vi "Write Scalar Data.vi"(8 "error in (no error)":errorcluster, 9 "Changed?":bool[](array[boolean]), 10 "Values":dbl[](array[numeric]), 11 "Cluster":T1 {"Data Type" format="%.0x"}) -> (0 "error out":errorcluster, 2 "Values":dbl[](array[numeric]), 3 "Cluster":T1 {"Data Type" format="%.0x"})   [LabVIEW 2016, in "FPGA Addon Engine.lvlib"]
uses:
  FPGA Addon Engine.lvlib
  Types/Register Settings.ctl
  Shared/Data Type.ctl
  Shared/Scalar Type.ctl
  <vilib>/rvi/errors/niLvFpgaAdjustHostInterfaceError.vi
  <vilib>/Utility/error.llb/Error Cluster From Error Code.vi
  <vilib>/rvi/interface/nirviReadWriteControl/nirviReadWriteControl.xnode
  <vilib>/rvi/interface/Simulation/niFpgaSimulationCallBeginRW.vi
  NiFpgaLv.dll
  Shared/FPGA Addon Shared.lvlib
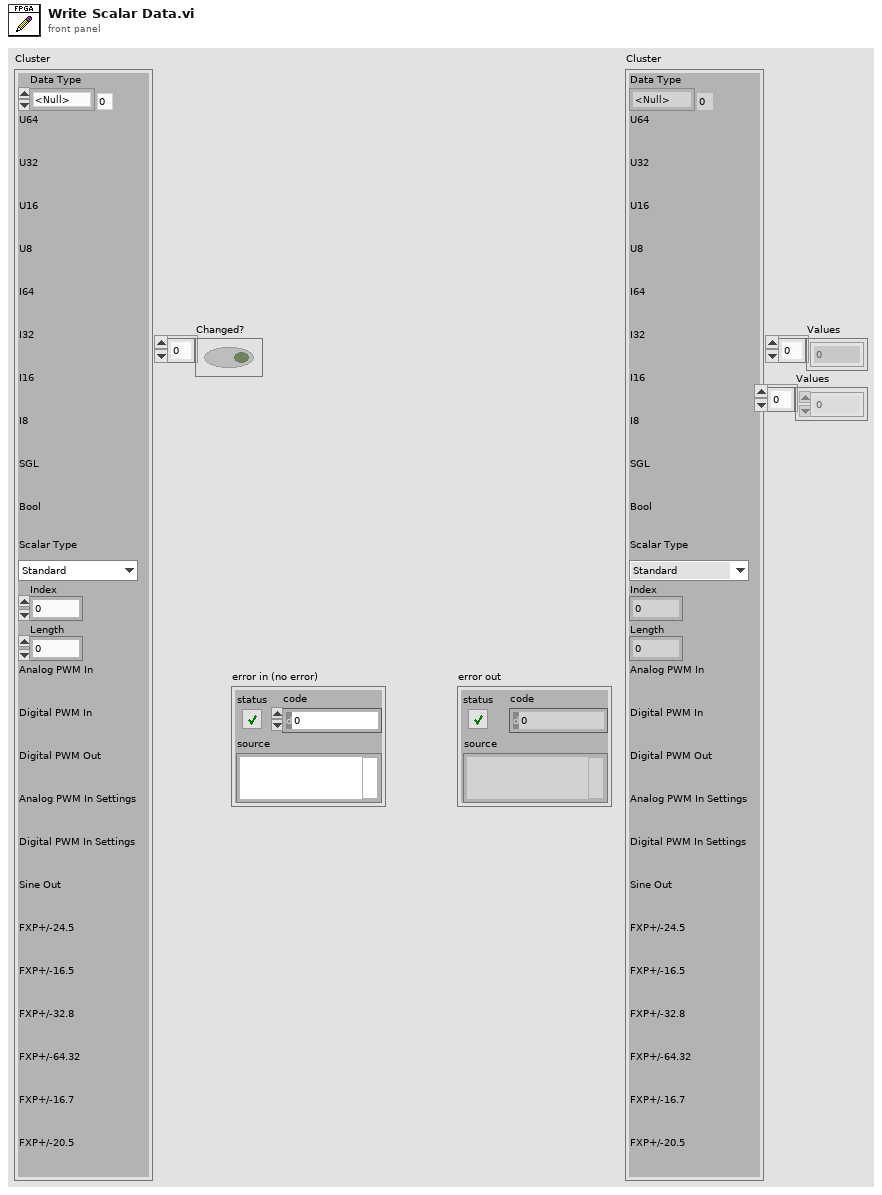
[diagram p1: front panel]
types:
  T1 = typedef "FPGA Addon Engine.lvlib/Register Settings.ctl" = cluster{"Data Type":T2, "U64":refnum<k20>, "U32":refnum<k20>, "U16":refnum<k20>, "U8":refnum<k20>, "I64":refnum<k20>, "I32":refnum<k20>, "I16":refnum<k20>, "I8":refnum<k20>, "SGL":refnum<k20>, "Bool":refnum<k20>, "Scalar Type":T3, "Index":i32, "Length":i32, "Analog PWM In":refnum<k20>, "Digital PWM In":refnum<k20>, "Digital PWM Out":refnum<k20>, "Analog PWM In Settings":refnum<k20>, "Digital PWM In Settings":refnum<k20>, "Sine Out":refnum<k20>, "FXP+/-24.5":refnum<k20>, "FXP+/-16.5":refnum<k20>, "FXP+/-32.8":refnum<k20>, "FXP+/-64.32":refnum<k20>, "FXP+/-16.7":refnum<k20>, "FXP+/-20.5":refnum<k20>}
  T2 = typedef "FPGA Addon Shared.lvlib/Data Type.ctl" = enum8{"<Null>", "I8", "I16", "I32", "I64", "U8", "U16", "U32", "U64", "SGL", "Boolean", "Analog PWM In Settings", "Analog PWM In", "Digital PWM In Settings", "Digital PWM In", "Digital PWM Out", "Sine Out", "FXP+/-24.5", "FXP+/-16.5", "FXP+/-32.8", "FXP+/-64.32", "FXP+/-16.7", "FXP+/-20.5"}
  T3 = typedef "FPGA Addon Shared.lvlib/Scalar Type.ctl" = enum16{"Standard", "Bitpacked"}
  T4 = cluster{"ACTIVE EDGE":bool, "TIMEOUT":u32, "THRESHOLD":fxp<+/-,32,8>}
  T5 = cluster{"ACTIVE EDGE":bool, "ACTIVE TICKS":u32, "INACTIVE TICKS":u32}
  T6 = cluster{"AMP":fxp<+/-,32,8>, "OFFSET":fxp<+/-,32,8>, "PERIODS/TICKS":fxp<+,32,0>}
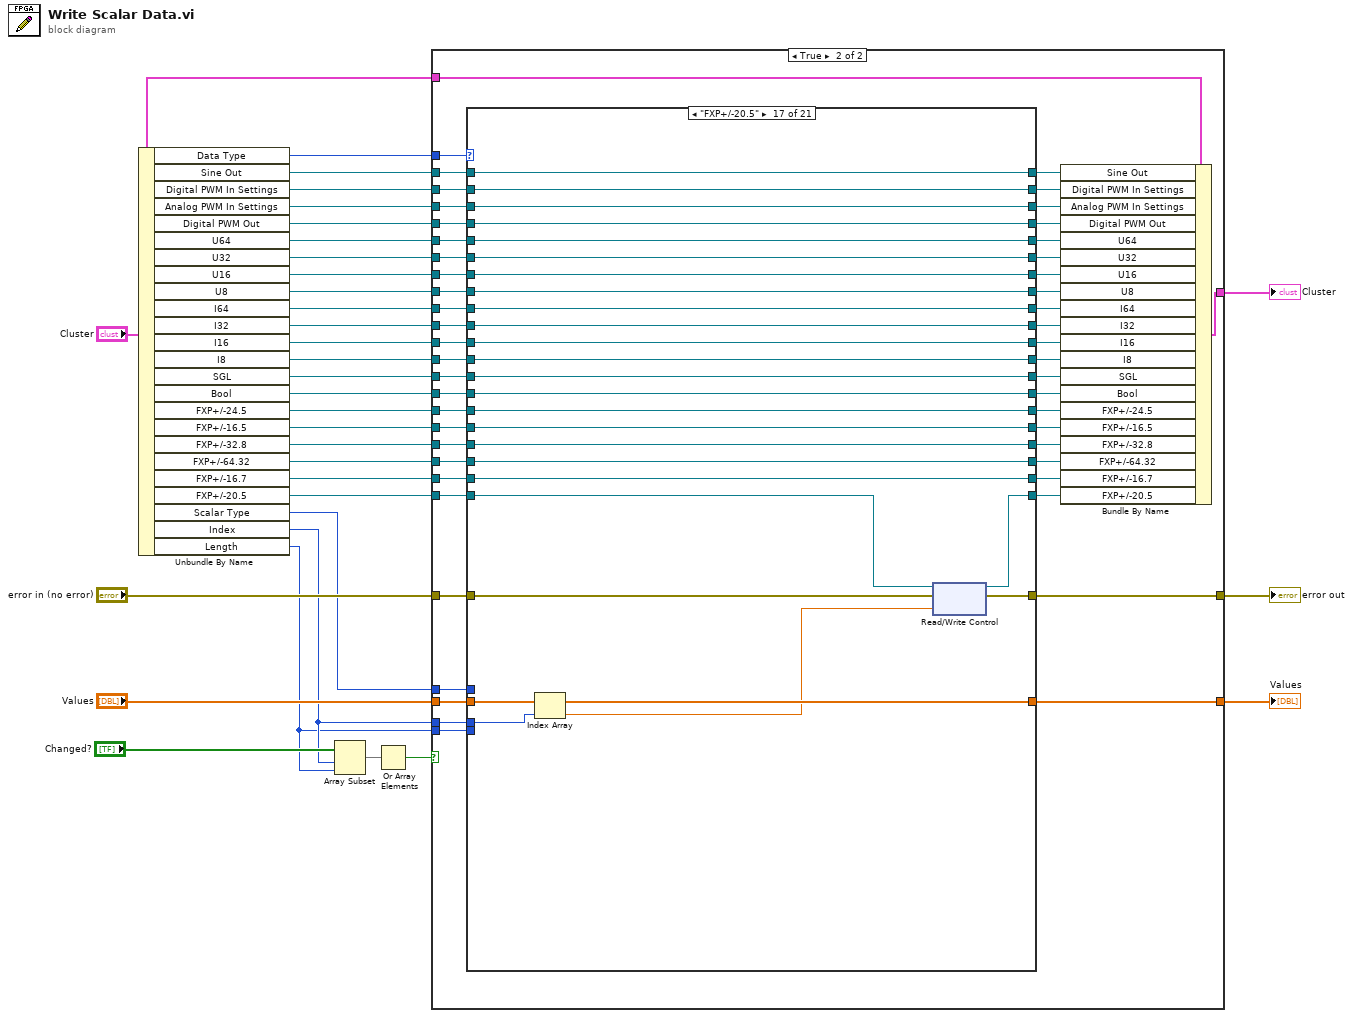
[diagram p0: block diagram]
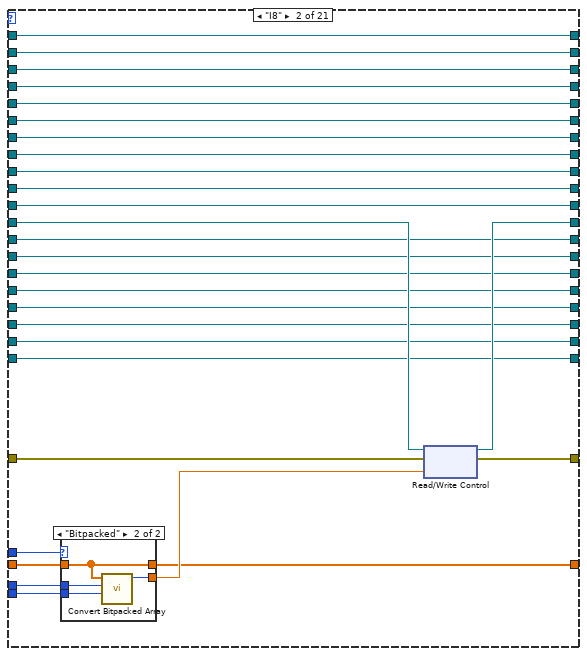
[diagram p4: hidden frame]
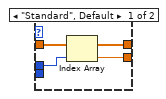
[diagram p5: hidden frame]
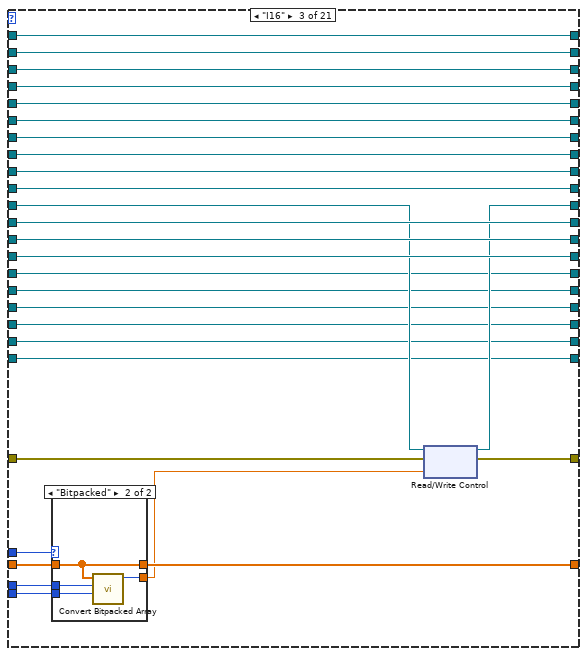
[diagram p6: hidden frame]
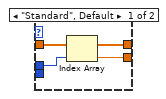
[diagram p7: hidden frame]
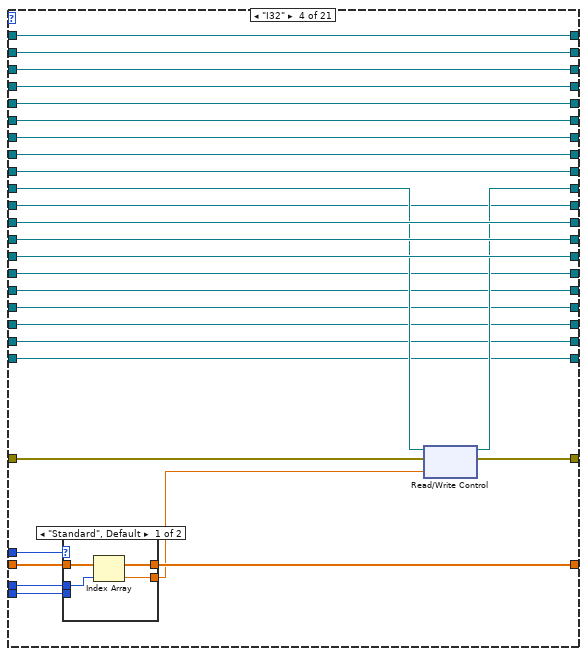
[diagram p8: hidden frame]
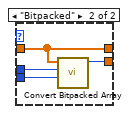
[diagram p9: hidden frame]
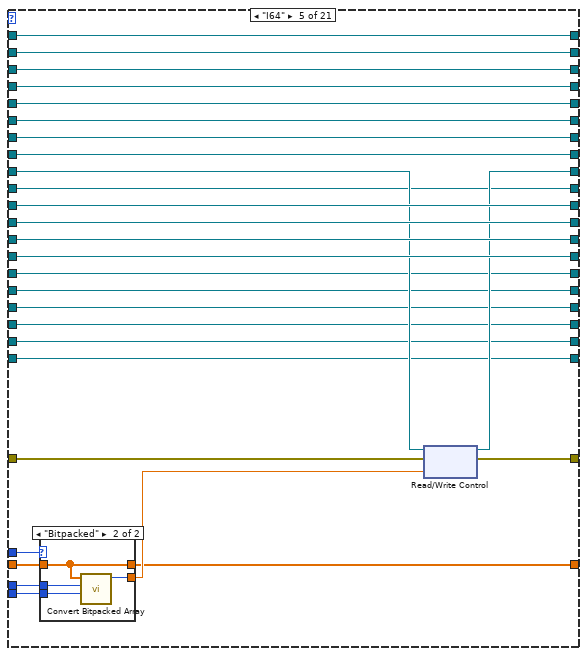
[diagram p10: hidden frame]
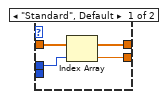
[diagram p11: hidden frame]
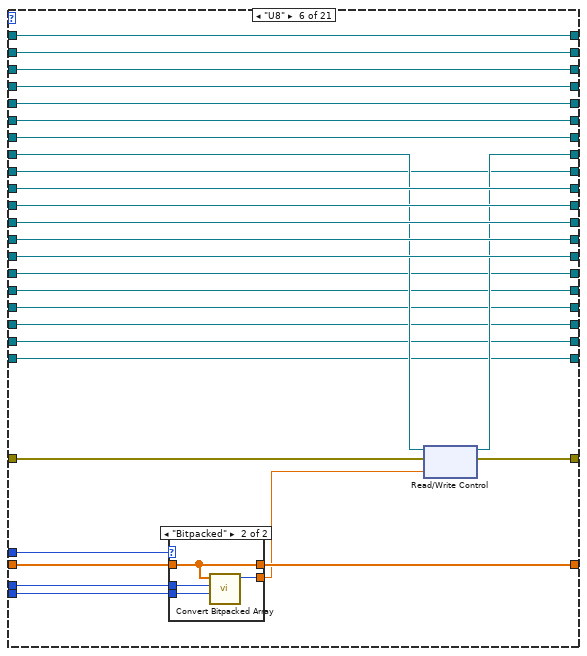
[diagram p12: hidden frame]
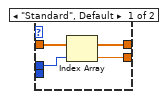
[diagram p13: hidden frame]
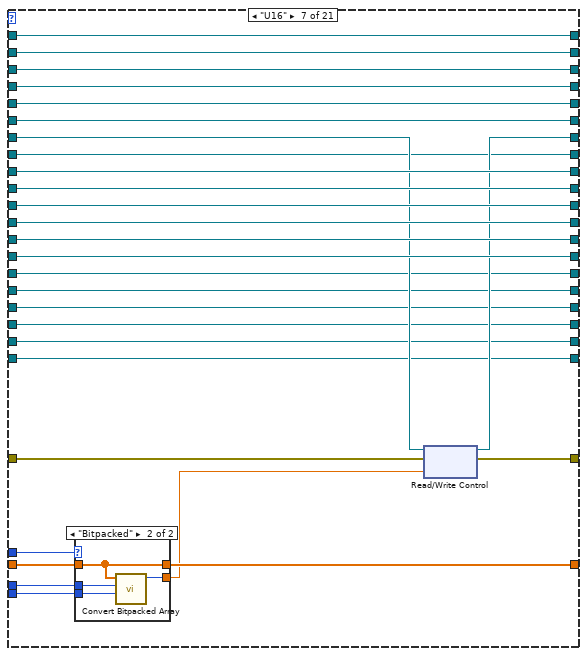
[diagram p14: hidden frame]
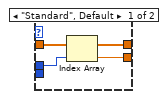
[diagram p15: hidden frame]
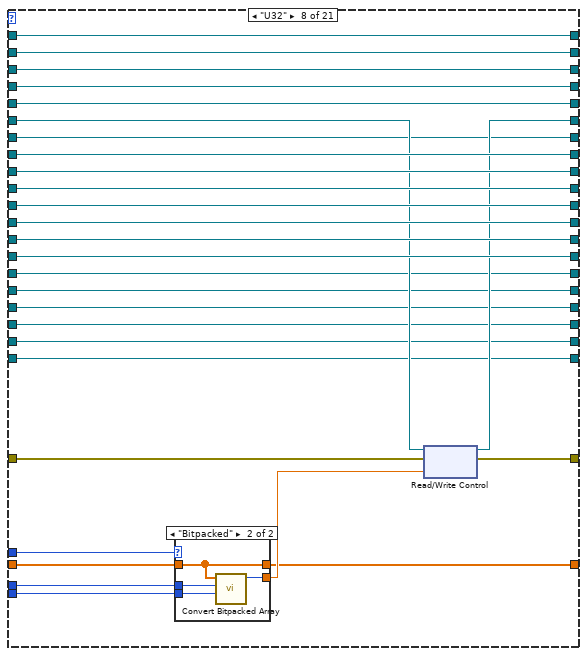
[diagram p16: hidden frame]
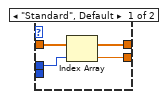
[diagram p17: hidden frame]
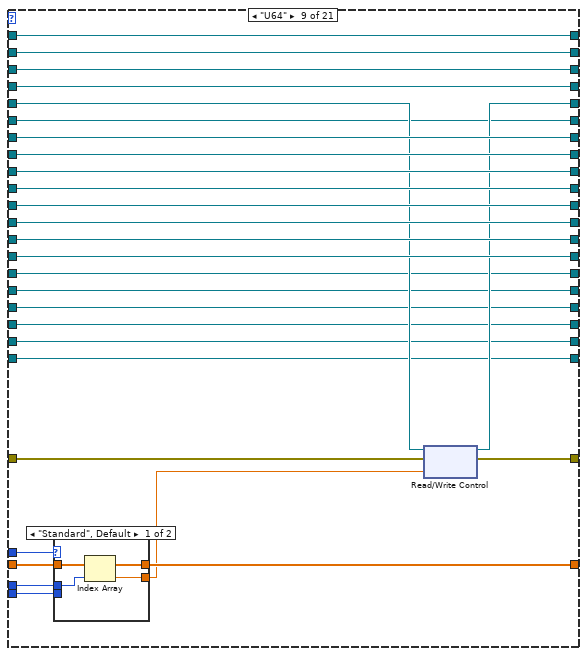
[diagram p18: hidden frame]
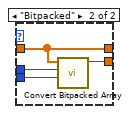
[diagram p19: hidden frame]
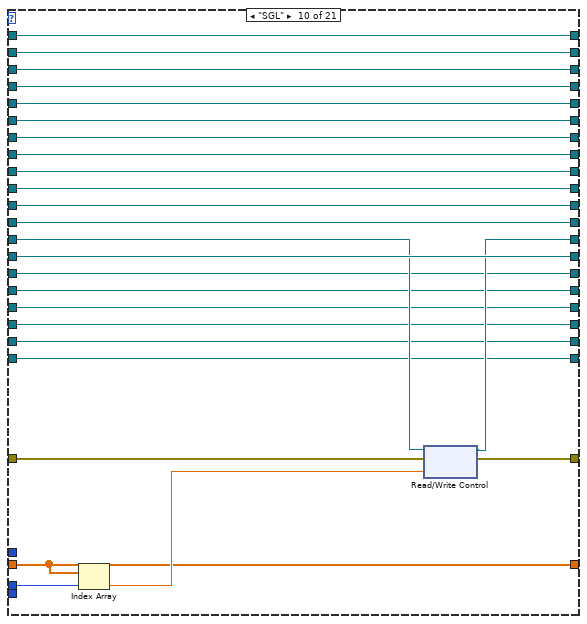
[diagram p20: hidden frame]
diagram:
  n1 = Unbundle By Name("Cluster") -> ("Data Type"=w33:T2, "Sine Out"=w7:refnum<k20>, "Digital PWM In Settings"=w13:refnum<k20>, "Analog PWM In Settings"=w14:refnum<k20>, "Digital PWM Out"=w15:refnum<k20>, "U64"=w20:refnum<k20>, "U32"=w21:refnum<k20>, "U16"=w22:refnum<k20>, "U8"=w23:refnum<k20>, "I64"=w24:refnum<k20>, "I32"=w25:refnum<k20>, "I16"=w26:refnum<k20>, "I8"=w32:refnum<k20>, "SGL"=w28:refnum<k20>, "Bool"=w27:refnum<k20>, "FXP+/-24.5"=w3:refnum<k20>, "FXP+/-16.5"=w4:refnum<k20>, "FXP+/-32.8"=w5:refnum<k20>, "FXP+/-64.32"=w6:refnum<k20>, "FXP+/-16.7"=w2:refnum<k20>, "FXP+/-20.5"=w1:refnum<k20>, "Scalar Type"=w16:T3, "Index"=w11:i32, "Length"=w10:i32)
  n2 = Array Subset(array="Changed?", index=w11, length=w10) -> (w9:bool[])
  n3 = Or Array Elements(Boolean array=w9) -> (logical OR=w8:bool)
  n4 = case shown="True" w8 {
    tunnel: w33 -> [_ w86]
    tunnel: w32 -> [_ w85]
    tunnel: "error in (no error)" -> [w35 w84]
    tunnel: [w35 w83] -> w30
    tunnel: "Cluster" -> [w36 w82]
    tunnel: w28 -> [_ w79]
    tunnel: w27 -> [_ w78]
    tunnel: w26 -> [_ w75]
    tunnel: w25 -> [_ w73]
    tunnel: w24 -> [_ w71]
    tunnel: w23 -> [_ w69]
    tunnel: w22 -> [_ w67]
    tunnel: w21 -> [_ w65]
    tunnel: w20 -> [_ w63]
    tunnel: [w36 w62] -> w19
    tunnel: [w34 w61] -> w18
    tunnel: "Values" -> [w34 w60]
    tunnel: w16 -> [_ w59]
    tunnel: w15 -> [_ w57]
    tunnel: w14 -> [_ w56]
    tunnel: w13 -> [_ w53]
    tunnel: w11 -> [_ w52]
    tunnel: w10 -> [_ w51]
    tunnel: w7 -> [_ w50]
    tunnel: w6 -> [_ w47]
    tunnel: w5 -> [_ w46]
    tunnel: w4 -> [_ w43]
    tunnel: w3 -> [_ w42]
    tunnel: w2 -> [_ w40]
    tunnel: w1 -> [_ w38]
    frame False {
    }
    frame True {
      n5 = case shown="\"FXP+/-20.5\"" w86 {
        tunnel: w85 -> [w106 w137 w163 w200 w237 w274 w311 w348 w385 w419 w448 w474 w500 w526 w552 w578 w604 w631 w665 w722 w759]
        tunnel: w84 -> [w98 w136 w173 w209 w245 w281 w317 w353 w389 w422 w450 w476 w502 w528 w554 w580 w606 w628 w662 w710 w747]
        tunnel: [w98 w135 w172 w208 w244 w280 w316 w352 w388 w421 w449 w475 w501 w527 w553 w579 w605 w627 w661 w709 w746] -> w83
        tunnel: [w106 w134 w163 w200 w237 w274 w311 w348 w385 w419 w448 w474 w500 w526 w552 w578 w604 w631 w665 w722 w759] -> w81
        tunnel: [w107 w133 w171 w207 w243 w279 w315 w351 w387 w410 w438 w466 w492 w518 w544 w570 w596 w630 w664 w721 w758] -> w80
        tunnel: w79 -> [w107 w133 w171 w207 w243 w279 w315 w351 w387 w412 w438 w466 w492 w518 w544 w570 w596 w630 w664 w721 w758]
        tunnel: w78 -> [w108 w132 w170 w206 w242 w278 w314 w350 w386 w420 w440 w455 w482 w509 w536 w562 w589 w629 w663 w720 w757]
        tunnel: [w108 w132 w170 w206 w242 w278 w314 w350 w386 w420 w439 w455 w482 w509 w536 w562 w589 w629 w663 w720 w757] -> w77
        tunnel: [w105 w131 w161 w197 w236 w273 w310 w347 w384 w418 w447 w473 w499 w525 w551 w577 w603 w632 w666 w719 w756] -> w76
        tunnel: w75 -> [w105 w131 w162 w197 w236 w273 w310 w347 w384 w418 w447 w473 w499 w525 w551 w577 w603 w632 w666 w719 w756]
        tunnel: [w104 w130 w169 w198 w233 w272 w309 w346 w383 w417 w446 w472 w498 w524 w550 w576 w602 w633 w667 w718 w755] -> w74
        tunnel: w73 -> [w104 w130 w169 w199 w233 w272 w309 w346 w383 w417 w446 w472 w498 w524 w550 w576 w602 w633 w667 w718 w755]
        tunnel: [w103 w129 w168 w205 w234 w269 w308 w345 w382 w416 w445 w471 w497 w523 w549 w575 w601 w634 w668 w717 w754] -> w72
        tunnel: w71 -> [w103 w129 w168 w205 w235 w269 w308 w345 w382 w416 w445 w471 w497 w523 w549 w575 w601 w634 w668 w717 w754]
        tunnel: [w102 w128 w167 w204 w241 w270 w305 w344 w381 w415 w444 w470 w496 w522 w548 w574 w600 w635 w669 w716 w753] -> w70
        tunnel: w69 -> [w102 w128 w167 w204 w241 w271 w305 w344 w381 w415 w444 w470 w496 w522 w548 w574 w600 w635 w669 w716 w753]
        tunnel: [w101 w127 w166 w203 w240 w277 w306 w341 w380 w414 w443 w469 w495 w521 w547 w573 w599 w636 w670 w715 w752] -> w68
        tunnel: w67 -> [w101 w127 w166 w203 w240 w277 w307 w341 w380 w414 w443 w469 w495 w521 w547 w573 w599 w636 w670 w715 w752]
        tunnel: [w100 w126 w165 w202 w239 w276 w313 w342 w377 w413 w442 w468 w494 w520 w546 w572 w598 w637 w671 w714 w751] -> w66
        tunnel: w65 -> [w100 w126 w165 w202 w239 w276 w313 w343 w377 w413 w442 w468 w494 w520 w546 w572 w598 w637 w671 w714 w751]
        tunnel: [w99 w125 w164 w201 w238 w275 w312 w349 w378 w411 w441 w467 w493 w519 w545 w571 w597 w638 w672 w713 w750] -> w64
        tunnel: w63 -> [w99 w125 w164 w201 w238 w275 w312 w349 w379 w411 w441 w467 w493 w519 w545 w571 w597 w638 w672 w713 w750]
        tunnel: [w97 w119 w156 w192 w227 w264 w300 w335 w372 w407 w435 w465 w491 w517 w543 w569 w595 w622 w658 w703 w745] -> w61
        tunnel: w60 -> [w97 w124 w160 w196 w232 w268 w304 w340 w376 w407 w435 w465 w491 w517 w543 w569 w595 w622 w658 w703 w745]
        tunnel: w51 -> [_ w122 w158 w193 w229 w267 w302 w338 w373 _ _ _ _ _ _ _ _ w623 w659 w702 w744]
        tunnel: w59 -> [_ w121 w157 w195 w231 w265 w301 w337 w375 _ _ _ _ _ _ _ _ _ _ _ _]
        tunnel: w52 -> [_ w123 w159 w194 w230 w266 w303 w339 w374 w409 w434 w464 w490 w516 w542 w568 w594 w624 w660 w701 w743]
        tunnel: [w96 w116 w152 w188 w224 w260 w296 w332 w368 w404 w430 w461 w487 w513 w539 w565 w591 w640 w673 w707 w739] -> w58
        tunnel: w57 -> [w96 w116 w152 w188 w224 w260 w296 w332 w368 w404 w430 w461 w487 w513 w539 w565 w591 w640 w673 w708 w739]
        tunnel: w56 -> [w95 w117 w153 w189 w225 w261 w297 w333 w369 w405 w431 w462 w488 w514 w540 w566 w592 w626 w652 w712 w749]
        tunnel: [w95 w117 w153 w189 w225 w261 w297 w333 w369 w405 w431 w462 w488 w514 w540 w566 w592 w625 w652 w712 w749] -> w55
        tunnel: [w94 w118 w154 w190 w226 w262 w298 w334 w370 w406 w432 w463 w489 w515 w541 w567 w593 w639 w654 w711 w748] -> w54
        tunnel: w53 -> [w94 w118 w154 w190 w226 w262 w298 w334 w370 w406 w432 w463 w489 w515 w541 w567 w593 w639 w653 w711 w748]
        tunnel: w50 -> [w93 w115 w151 w187 w223 w259 w295 w331 w367 w403 w429 w460 w486 w512 w538 w564 w590 w615 w649 w682 w741]
        tunnel: [w93 w115 w151 w187 w223 w259 w295 w331 w367 w403 w429 w460 w486 w512 w538 w564 w590 w615 w649 w682 w740] -> w49
        tunnel: [w92 w114 w150 w186 w222 w258 w294 w330 w366 w402 w428 w459 w485 w511 w531 w558 w585 w614 w646 w679 w731] -> w48
        tunnel: w47 -> [w92 w114 w150 w186 w222 w258 w294 w330 w366 w402 w428 w459 w485 w511 w533 w558 w585 w614 w646 w679 w731]
        tunnel: w46 -> [w91 w113 w149 w185 w221 w257 w293 w329 w365 w401 w427 w458 w484 w505 w532 w559 w586 w613 w645 w678 w730]
        tunnel: [w91 w113 w149 w185 w221 w257 w293 w329 w365 w401 w427 w458 w484 w506 w532 w559 w586 w613 w645 w678 w730] -> w45
        tunnel: [w90 w112 w148 w184 w220 w256 w292 w328 w364 w400 w426 w457 w479 w507 w534 w560 w587 w612 w644 w677 w729] -> w44
        tunnel: w43 -> [w90 w112 w148 w184 w220 w256 w292 w328 w364 w400 w426 w457 w480 w507 w534 w560 w587 w612 w644 w677 w729]
        tunnel: w42 -> [w89 w111 w147 w183 w219 w255 w291 w327 w363 w399 w425 w454 w481 w508 w535 w561 w588 w611 w643 w676 w728]
        tunnel: [w89 w111 w147 w183 w219 w255 w291 w327 w363 w399 w425 w453 w481 w508 w535 w561 w588 w611 w643 w676 w728] -> w41
        tunnel: w40 -> [w88 w110 w146 w182 w218 w254 w290 w326 w362 w398 w424 w452 w478 w504 w530 w557 w583 w610 w642 w675 w727]
        tunnel: [w88 w110 w146 w182 w218 w254 w290 w326 w362 w398 w424 w452 w478 w504 w530 w556 w583 w610 w642 w675 w727] -> w39
        tunnel: w38 -> [w87 w109 w145 w181 w217 w253 w289 w325 w361 w397 w423 w451 w477 w503 w529 w555 w584 w607 w641 w674 w726]
        tunnel: [w87 w109 w145 w181 w217 w253 w289 w325 w361 w397 w423 w451 w477 w503 w529 w555 w582 w607 w641 w674 w726] -> w37
        frame "<Null>", Default {
        }
        frame "I8" {
          n6 = case shown="\"Bitpacked\"" w121 {
            tunnel: w124 -> [w138 w141]
            tunnel: w123 -> [w140 w144]
            tunnel: [w139 w142] -> w120
            tunnel: w122 -> [_ w143]
            tunnel: [w138 w141] -> w119
            frame "Standard", Default {
              n7 = Index Array(array=w138, index=w140) -> (element=w139:dbl)
            }
            frame "Bitpacked" {
              n8 = call "Convert Bitpacked Array.vi"("Length"=w143, "Index"=w144, "Values"=w141) -> ("Numeric"=w142:u64)  [unwired: 8 in]
            }
          }
          n9 = xnode "Read/Write Control"("FPGA VI Reference In"=w137, "error in"=w136, "Value"=w120) -> ("FPGA VI Reference Out"=w134:refnum<k20>, "error out"=w135:errorcluster)
        }
        frame "I16" {
          n10 = case shown="\"Bitpacked\"" w157 {
            tunnel: w160 -> [w174 w177]
            tunnel: w159 -> [w176 w180]
            tunnel: [w175 w178] -> w155
            tunnel: w158 -> [_ w179]
            tunnel: [w174 w177] -> w156
            frame "Standard", Default {
              n11 = Index Array(array=w174, index=w176) -> (element=w175:dbl)
            }
            frame "Bitpacked" {
              n12 = call "Convert Bitpacked Array.vi"("Length"=w179, "Index"=w180, "Values"=w177) -> ("Numeric"=w178:u64)  [unwired: 8 in]
            }
          }
          n13 = xnode "Read/Write Control"("FPGA VI Reference In"=w162, "error in"=w173, "Value"=w155) -> ("FPGA VI Reference Out"=w161:refnum<k20>, "error out"=w172:errorcluster)
        }
        frame "I32" {
          n14 = case shown="\"Standard\", Default" w195 {
            tunnel: w196 -> [w210 w213]
            tunnel: w194 -> [w212 w216]
            tunnel: [w211 w214] -> w191
            tunnel: w193 -> [_ w215]
            tunnel: [w210 w213] -> w192
            frame "Standard", Default {
              n15 = Index Array(array=w210, index=w212) -> (element=w211:dbl)
            }
            frame "Bitpacked" {
              n16 = call "Convert Bitpacked Array.vi"("Length"=w215, "Index"=w216, "Values"=w213) -> ("Numeric"=w214:u64)  [unwired: 8 in]
            }
          }
          n17 = xnode "Read/Write Control"("FPGA VI Reference In"=w199, "error in"=w209, "Value"=w191) -> ("FPGA VI Reference Out"=w198:refnum<k20>, "error out"=w208:errorcluster)
        }
        frame "I64" {
          n18 = case shown="\"Bitpacked\"" w231 {
            tunnel: w232 -> [w246 w249]
            tunnel: w230 -> [w248 w252]
            tunnel: [w247 w250] -> w228
            tunnel: w229 -> [_ w251]
            tunnel: [w246 w249] -> w227
            frame "Standard", Default {
              n19 = Index Array(array=w246, index=w248) -> (element=w247:dbl)
            }
            frame "Bitpacked" {
              n20 = call "Convert Bitpacked Array.vi"("Length"=w251, "Index"=w252, "Values"=w249) -> ("Numeric"=w250:u64)  [unwired: 8 in]
            }
          }
          n21 = xnode "Read/Write Control"("FPGA VI Reference In"=w235, "error in"=w245, "Value"=w228) -> ("FPGA VI Reference Out"=w234:refnum<k20>, "error out"=w244:errorcluster)
        }
        frame "U8" {
          n22 = case shown="\"Bitpacked\"" w265 {
            tunnel: w268 -> [w282 w285]
            tunnel: w266 -> [w284 w288]
            tunnel: [w283 w286] -> w263
            tunnel: w267 -> [_ w287]
            tunnel: [w282 w285] -> w264
            frame "Standard", Default {
              n23 = Index Array(array=w282, index=w284) -> (element=w283:dbl)
            }
            frame "Bitpacked" {
              n24 = call "Convert Bitpacked Array.vi"("Length"=w287, "Index"=w288, "Values"=w285) -> ("Numeric"=w286:u64)  [unwired: 8 in]
            }
          }
          n25 = xnode "Read/Write Control"("FPGA VI Reference In"=w271, "error in"=w281, "Value"=w263) -> ("FPGA VI Reference Out"=w270:refnum<k20>, "error out"=w280:errorcluster)
        }
        frame "U16" {
          n26 = case shown="\"Bitpacked\"" w301 {
            tunnel: w304 -> [w318 w321]
            tunnel: w303 -> [w320 w324]
            tunnel: [w319 w322] -> w299
            tunnel: w302 -> [_ w323]
            tunnel: [w318 w321] -> w300
            frame "Standard", Default {
              n27 = Index Array(array=w318, index=w320) -> (element=w319:dbl)
            }
            frame "Bitpacked" {
              n28 = call "Convert Bitpacked Array.vi"("Length"=w323, "Index"=w324, "Values"=w321) -> ("Numeric"=w322:u64)  [unwired: 8 in]
            }
          }
          n29 = xnode "Read/Write Control"("FPGA VI Reference In"=w307, "error in"=w317, "Value"=w299) -> ("FPGA VI Reference Out"=w306:refnum<k20>, "error out"=w316:errorcluster)
        }
        frame "U32" {
          n30 = case shown="\"Bitpacked\"" w337 {
            tunnel: w340 -> [w354 w357]
            tunnel: w339 -> [w356 w360]
            tunnel: [w355 w358] -> w336
            tunnel: w338 -> [_ w359]
            tunnel: [w354 w357] -> w335
            frame "Standard", Default {
              n31 = Index Array(array=w354, index=w356) -> (element=w355:dbl)
            }
            frame "Bitpacked" {
              n32 = call "Convert Bitpacked Array.vi"("Length"=w359, "Index"=w360, "Values"=w357) -> ("Numeric"=w358:u64)  [unwired: 8 in]
            }
          }
          n33 = xnode "Read/Write Control"("FPGA VI Reference In"=w343, "error in"=w353, "Value"=w336) -> ("FPGA VI Reference Out"=w342:refnum<k20>, "error out"=w352:errorcluster)
        }
        frame "U64" {
          n34 = case shown="\"Standard\", Default" w375 {
            tunnel: w376 -> [w390 w393]
            tunnel: w374 -> [w392 w396]
            tunnel: [w391 w394] -> w371
            tunnel: w373 -> [_ w395]
            tunnel: [w390 w393] -> w372
            frame "Standard", Default {
              n35 = Index Array(array=w390, index=w392) -> (element=w391:dbl)
            }
            frame "Bitpacked" {
              n36 = call "Convert Bitpacked Array.vi"("Length"=w395, "Index"=w396, "Values"=w393) -> ("Numeric"=w394:u64)  [unwired: 8 in]
            }
          }
          n37 = xnode "Read/Write Control"("FPGA VI Reference In"=w379, "error in"=w389, "Value"=w371) -> ("FPGA VI Reference Out"=w378:refnum<k20>, "error out"=w388:errorcluster)
        }
        frame "SGL" {
          n38 = Index Array(array=w407, index=w409) -> (element=w408:dbl)
          n39 = xnode "Read/Write Control"("FPGA VI Reference In"=w412, "error in"=w422, "Value"=w408) -> ("FPGA VI Reference Out"=w410:refnum<k20>, "error out"=w421:errorcluster)
        }
        frame "Boolean" {
          n40 = Index Array(array=w435, index=w434) -> (element=w433:dbl)
          n41 = To Unsigned Byte Integer(number=w433) -> (unsigned 8bit integer=w436:u8)
          n42 = Greater Than 0?(x=w436) -> (x > 0?=w437:bool)
          n43 = xnode "Read/Write Control"("FPGA VI Reference In"=w440, "error in"=w450, "Value"=w437) -> ("FPGA VI Reference Out"=w439:refnum<k20>, "error out"=w449:errorcluster)
        }
        frame "FXP+/-24.5" {
          n44 = Index Array(array=w465, index=w464) -> (element=w456:dbl)
          n45 = xnode "Read/Write Control"("FPGA VI Reference In"=w454, "error in"=w476, "Value"=w456) -> ("FPGA VI Reference Out"=w453:refnum<k20>, "error out"=w475:errorcluster)
        }
        frame "FXP+/-16.5" {
          n46 = Index Array(array=w491, index=w490) -> (element=w483:dbl)
          n47 = xnode "Read/Write Control"("FPGA VI Reference In"=w480, "error in"=w502, "Value"=w483) -> ("FPGA VI Reference Out"=w479:refnum<k20>, "error out"=w501:errorcluster)
        }
        frame "FXP+/-32.8" {
          n48 = Index Array(array=w517, index=w516) -> (element=w510:dbl)
          n49 = xnode "Read/Write Control"("FPGA VI Reference In"=w505, "error in"=w528, "Value"=w510) -> ("FPGA VI Reference Out"=w506:refnum<k20>, "error out"=w527:errorcluster)
        }
        frame "FXP+/-64.32" {
          n50 = Index Array(array=w543, index=w542) -> (element=w537:dbl)
          n51 = xnode "Read/Write Control"("FPGA VI Reference In"=w533, "error in"=w554, "Value"=w537) -> ("FPGA VI Reference Out"=w531:refnum<k20>, "error out"=w553:errorcluster)
        }
        frame "FXP+/-16.7" {
          n52 = Index Array(array=w569, index=w568) -> (element=w563:dbl)
          n53 = xnode "Read/Write Control"("FPGA VI Reference In"=w557, "error in"=w580, "Value"=w563) -> ("FPGA VI Reference Out"=w556:refnum<k20>, "error out"=w579:errorcluster)
        }
        frame "FXP+/-20.5" {
          n54 = Index Array(array=w595, index=w594) -> (element=w581:dbl)
          n55 = xnode "Read/Write Control"("FPGA VI Reference In"=w584, "error in"=w606, "Value"=w581) -> ("FPGA VI Reference Out"=w582:refnum<k20>, "error out"=w605:errorcluster)
        }
        frame "Analog PWM In Settings" {
          n56 = Array Subset(array=w622, index=w624, length=w623) -> (w621:dbl[])
          n57 = Index Array(array=w621) -> (element #1=w619:dbl, element #2=w617:dbl, element #3=w616:dbl)  [unwired: 4 in, 1 out]
          n58 = Greater?(x=w619, y=0.5) -> (0:w618:bool)
          n59 = Bundle By Name(cluster=T4 {"ACTIVE EDGE"=FALSE, "TIMEOUT"=0, "THRESHOLD"=0.0} ("Value"), "ACTIVE EDGE"=w618, "TIMEOUT"=w617, "THRESHOLD"=w616) -> (w608:T4)
          n60 = xnode "Read/Write Control"("FPGA VI Reference In"=w626, "error in"=w628, "Value"=w608) -> ("FPGA VI Reference Out"=w625:refnum<k20>, "error out"=w627:errorcluster)
        }
        frame "Digital PWM In Settings" {
          n61 = Array Subset(array=w658, index=w660, length=w659) -> (w657:dbl[])
          n62 = Index Array(array=w657) -> (element #1=w651:dbl, element #2=w650:dbl)  [unwired: 2 in]
          n63 = Greater?(x=w651, y=0.5) -> (0:w656:bool)
          n64 = Bundle By Name(cluster=cluster{"ACTIVE EDGE":bool, "TIMEOUT":u32} {"ACTIVE EDGE"=FALSE, "TIMEOUT"=0} ("Value"), "ACTIVE EDGE"=w656, "TIMEOUT"=w650) -> (w647:cluster{"ACTIVE EDGE":bool, "TIMEOUT":u32})
          n65 = xnode "Read/Write Control"("FPGA VI Reference In"=w653, "error in"=w662, "Value"=w647) -> ("FPGA VI Reference Out"=w654:refnum<k20>, "error out"=w661:errorcluster)
        }
        frame "Digital PWM Out" {
          n66 = Array Subset(array=w703, index=w701, length=w702) -> (w700:dbl[])
          n67 = Index Array(array=w700) -> (element #1=w695:dbl, element #2=w693:dbl, element #3=w694:dbl)  [unwired: 3 in]
          n68 = To Single Precision Float(number=w693) -> (single precision float=w687:sgl)
          n69 = To Single Precision Float(number=w694) -> (single precision float=w686:sgl)
          n70 = In Range and Coerce(upper limit=sgl 100.0, x=w686, lower limit=sgl 0.0) -> (coerced(x)=w685:sgl)  [unwired: 1 out]
          n71 = Equal To 0?(x=w687) -> (x = 0?=w692:bool)
          n72 = Divide(x=sgl 40000000.0 ("y"), y=w687) -> (x/y=w690:sgl)
          n73 = Multiply(x=w685, y=sgl 0.01 ("x")) -> (x*y=w688:sgl)
          n74 = case shown="True" w692 {
            tunnel: [w724 w725] -> w691
            tunnel: w690 -> [w724 _]
            tunnel: [w723 w725] -> w689
            tunnel: w688 -> [w723 _]
            frame False {
            }
            frame True {
              w725 = sgl 0.0
            }
          }
          n75 = Greater?(x=w695, y=0.5) -> (0:w698:bool)
          n76 = To Unsigned Long Integer(number=w691) -> (unsigned 32bit integer=w705:u32)
          n77 = Multiply(x=w691, y=w689) -> (x*y=w697:u32)
          n78 = Subtract(x=w705, y=w697) -> (x-y=w696:u32)
          n79 = Bundle By Name(cluster=T5 {"ACTIVE EDGE"=FALSE, "ACTIVE TICKS"=0, "INACTIVE TICKS"=0} ("Value"), "ACTIVE EDGE"=w698, "ACTIVE TICKS"=w697, "INACTIVE TICKS"=w696) -> (w680:T5)
          n80 = xnode "Read/Write Control"("FPGA VI Reference In"=w708, "error in"=w710, "Value"=w680) -> ("FPGA VI Reference Out"=w707:refnum<k20>, "error out"=w709:errorcluster)
        }
        frame "Sine Out" {
          n81 = Array Subset(array=w745, index=w743, length=w744) -> (w742:dbl[])
          n82 = Index Array(array=w742) -> (element #1=w735:dbl, element #2=w736:dbl, element #3=w737:dbl)  [unwired: 3 in]
          n83 = Divide(x=w737, y=sgl 40000000.0) -> (x/y=w734:dbl)
          n84 = Bundle By Name(cluster=T6 {"AMP"=0.0, "OFFSET"=0.0, "PERIODS/TICKS"=0.0} ("Value"), "AMP"=w735, "OFFSET"=w736, "PERIODS/TICKS"=w734) -> (w732:T6)
          n85 = xnode "Read/Write Control"("FPGA VI Reference In"=w741, "error in"=w747, "Value"=w732) -> ("FPGA VI Reference Out"=w740:refnum<k20>, "error out"=w746:errorcluster)
        }
      }
      n86 = Bundle By Name(cluster=w82, "Sine Out"=w49, "Digital PWM In Settings"=w54, "Analog PWM In Settings"=w55, "Digital PWM Out"=w58, "U64"=w64, "U32"=w66, "U16"=w68, "U8"=w70, "I64"=w72, "I32"=w74, "I16"=w76, "I8"=w81, "SGL"=w80, "Bool"=w77, "FXP+/-24.5"=w41, "FXP+/-16.5"=w44, "FXP+/-32.8"=w45, "FXP+/-64.32"=w48, "FXP+/-16.7"=w39, "FXP+/-20.5"=w37) -> (w62:T1)
    }
  }
  "error out" <- w30
  "Cluster" <- w19
  "Values" <- w18
